vi "subVI for sorting.vi"(9 "identifier":string, 10 "string":string) -> (0 "moving\naverage":waveform(i64), 1 "output":waveform(i64), 2 "has input":bool)   [LabVIEW 2012]
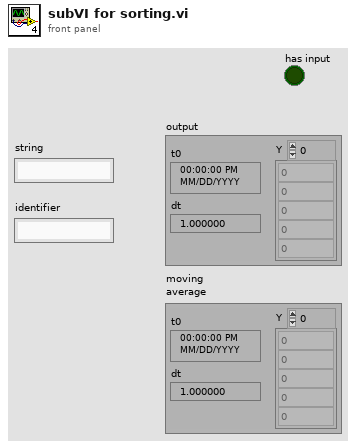
[diagram p1: front panel]
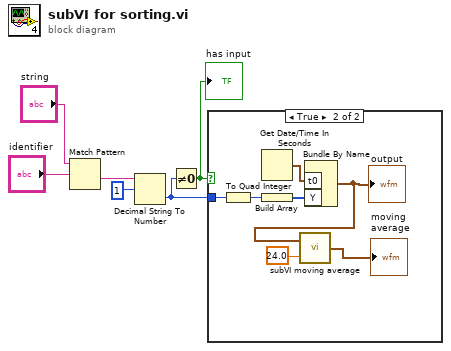
[diagram p0: block diagram]
diagram:
  n1 = Match Pattern(string="string", regular expression="identifier") -> (after substring=w2:string)  [unwired: 1 in, 3 out]
  n2 = Decimal String To Number(string=w2, offset=1) -> (number=w4:i32)  [unwired: 1 in, 1 out]
  n3 = Not Equal To 0?(x=w4) -> (x != 0?=w5:bool)
  "has input" <- w5
  n4 = case shown="True" w5 {
    tunnel: w4 -> [_ w10]
    frame False {
    }
    frame True {
      n5 = To Quad Integer(1:w10) -> (0:w12:i64)
      n6 = Get Date/Time In Seconds() -> (seconds since 1Jan1904=w13:timestamp)
      n7 = Build Array(w12) -> (w11:i64[])
      n8 = Bundle By Name("t0"=w13, "Y"=w11) -> (w7:waveform(i64))  [unwired: 1 in]
      "output" <- w7
      n9 = call "subVI moving average.vi"("lenght"=24.0, "input"=w7) -> ("output"=→"moving\naverage":waveform(i64))  [unwired: 1 in]
    }
  }
